vi "Down Shift Commanded.vi"(8 "error in":errorcluster) -> (0 "error out":errorcluster, 3 "Down Shift Commanded":bool)   [LabVIEW 2015]
uses:
  Support/Global Objects.vi
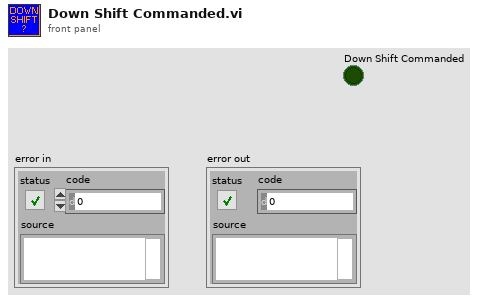
[diagram p1: front panel]
types:
  T1 = typedef "Teleop Commands.ctl" = cluster{"Throttle":dbl, "Turn":dbl, "Up Shift Commanded":bool, "Down Shift Commanded":bool}
  T2 = typedef "Configuration.ctl" = cluster{"Throttle Dead Zone":dbl, "Throttle Ramp Rate":dbl, "Turn Dead Zone":dbl, "Auton":cluster{"Motion Plan P":dbl, "Motion Plan I":dbl, "Motion Plan D":dbl}, "Auto Upshift Enabled":bool, "Upshift Min Throttle":dbl, "Upshift Min Velocity":dbl, "Min time before upshift":dbl, "Shift Throttle Detent":u32, "Min time before downshift":dbl, "Turn PID":cluster{"Motion Plan P":dbl, "Motion Plan I":dbl, "Motion Plan D":dbl}, "Auto Coast Downshift":bool, "Downshift Coast Max Vel":dbl, "Downshift Coast Throttle Epsilon":dbl}
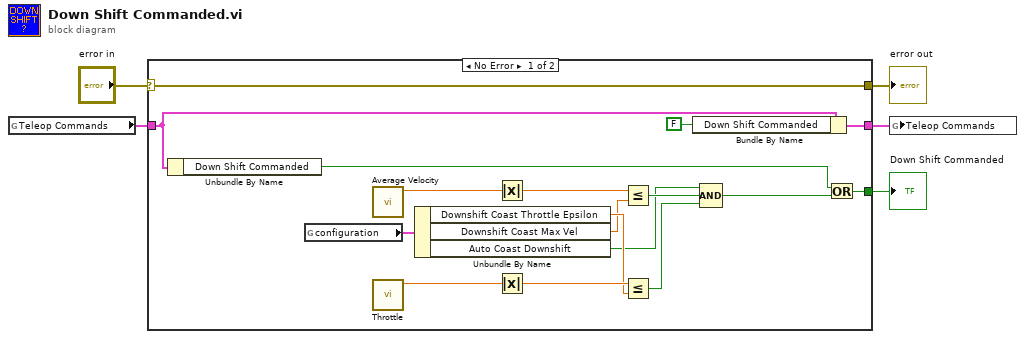
[diagram p0: block diagram]
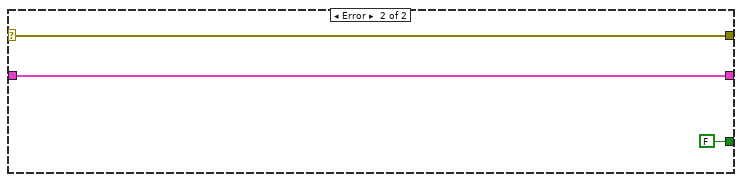
[diagram p2: hidden frame]
diagram:
  n1 = global read "Global Objects.vi" "Teleop Commands"() -> (w3:T1)
  n2 = case shown="No Error" "error in" {
    selector: "error in" -> [w22 w25]
    tunnel: [w22 w25] -> w4
    tunnel: [w20 w24] -> w2
    tunnel: w3 -> [w21 w24]
    tunnel: [w6 FALSE ("Up Shift Commanded")] -> w1
    frame No Error {
      n3 = Unbundle By Name(w21) -> ("Down Shift Commanded"=w7:bool)
      n4 = global read "Global Objects.vi" "configuration"() -> (w16:T2)
      n5 = call "Average Velocity.vi"() -> ("Average Velocity"=w17:dbl)  [unwired: 11 in]
      n6 = call "Throttle.vi"() -> ("throttle"=w18:dbl)  [unwired: 10 in, 1 out]
      n7 = Unbundle By Name(w16) -> ("Downshift Coast Throttle Epsilon"=w14:dbl, "Downshift Coast Max Vel"=w10:dbl, "Auto Coast Downshift"=w9:bool)
      n8 = Absolute Value(x=w17) -> (abs(x)=w11:dbl)
      n9 = Absolute Value(x=w18) -> (abs(x)=w15:dbl)
      n10 = Less Or Equal?(x=w11, y=w10) -> (x <= y?=w13:bool)
      n11 = Less Or Equal?(x=w15, y=w14) -> (x <= y?=w12:bool)
      n12 = Bundle By Name(cluster=w21, "Down Shift Commanded"=FALSE ("Up Shift Commanded")) -> (w20:T1)
      n13 = Compound Arithmetic op=AND(w9, w13, w12) -> (w8:bool)
      n14 = Or(x=w7, y=w8) -> (x .or. y?=w6:bool)
    }
    frame Error {
    }
  }
  "error out" <- w4
  "Down Shift Commanded" <- w1
  n15 = global write "Global Objects.vi" "Teleop Commands"(w2) -> ()
